vi "数组.vi"() -> ()   [LabVIEW 2012]
panel:
  out "大小 2":i32
  out "数组 2":dbl[](array[numeric])
  out "大小":i32
  out "数组":dbl[](array[numeric])
  out "波形图":dbl[](graph)
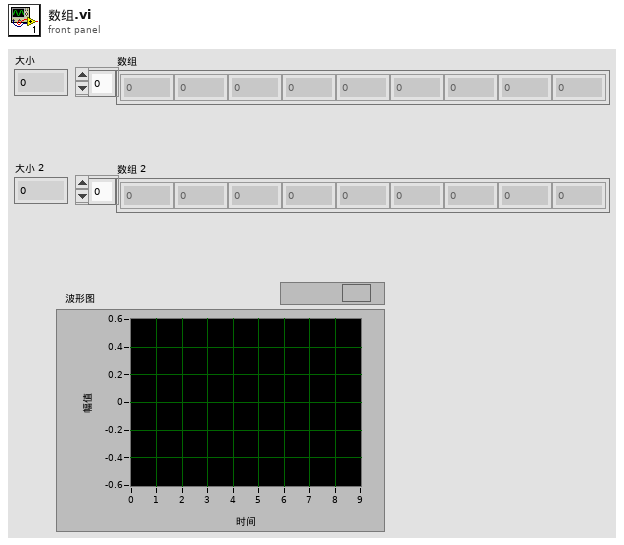
[diagram p1: front panel]
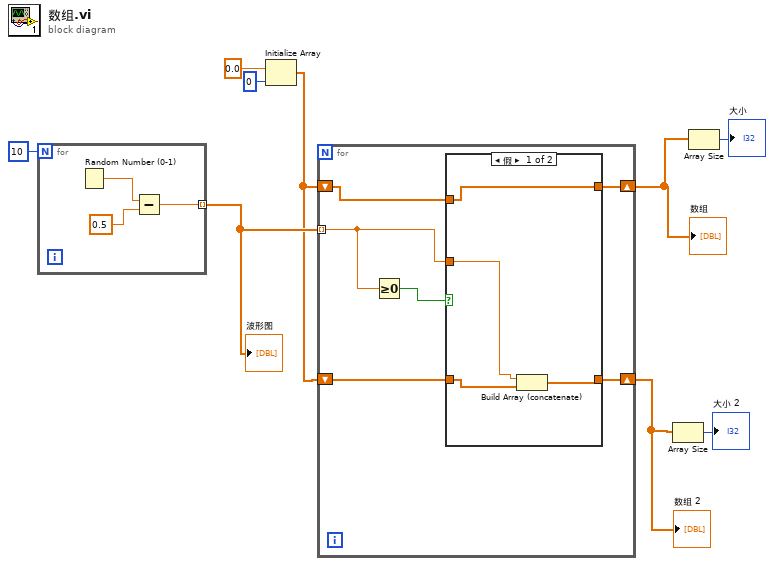
[diagram p0: block diagram]
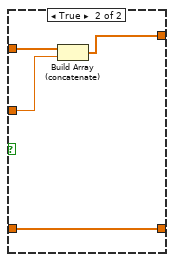
[diagram p2: hidden frame]
diagram:
  n1 = for {
    N: 10 -> [_]
    tunnel: [w10] -> w8 mode=indexing
    n2 = Random Number (0-1)() -> (number: 0 to 1=w12:dbl)
    n3 = Subtract(x=w12, y=0.5) -> (x-y=w10:dbl)
  }
  "波形图" <- w8
  n4 = Initialize Array(0.0 ("元素"), 0 ("维数大小")) -> (w2:dbl[])
  n5 = for {
    tunnel: w8 -> [w17] mode=indexing
    shift-right: [w15] -> w4
    shift-left: w2 -> [w16]
    shift-right: [w14] -> w1
    shift-left: w2 -> [w13]
    n6 = Greater Or Equal To 0?(x=w17) -> (x >= 0?=w18:bool)
    n7 = case shown="假" w18 {
      tunnel: w17 -> [w20 w26]
      tunnel: w16 -> [w21 w25]
      tunnel: [w21 w24] -> w15
      tunnel: [w19 w23] -> w14
      tunnel: w13 -> [w22 w23]
      frame False {
        n8 = Build Array (concatenate)(w20, w22) -> (w19:dbl[])
      }
      frame True {
        n9 = Build Array (concatenate)(w25, w26) -> (w24:dbl[])
      }
    }
  }
  "数组" <- w4
  "数组 2" <- w1
  n10 = Array Size(array=w1) -> (size(s)=→"大小 2":i32)
  n11 = Array Size(array=w4) -> (size(s)=→"大小":i32)
